vi "Bloco_escritaSuper.vi"(0 "reference":refnum<vi>, 1 "error in (no error)":errorcluster, 2 "Tag_para_PDF":string, 3 "Tipo de Dado":T6 items=["Engenharia", "Puro(mA)"], 4 "Abrir Editor Prioridade":bool, 7 "todos_os_dados_SAIDA":T1) -> (14 "reference out":refnum<vi>, 15 "error out":errorcluster)   [LabVIEW 2019]
uses:
  \\SERVERPC\Server/padrao_tipo_dado.ctl
  \\SERVERPC\Server/padrao_todos_os_dados_SAIDA.ctl
  \\SERVERPC\Server/padrao_UCM.004.EEL.0300_SAIDA.ctl
  \\SERVERPC\Server/padrao_UCM.004.EEL.0200_SAIDA.ctl
  \\SERVERPC\Server/padrao_INTERNO.ctl
  \\SERVERPC\Server/padrao_ADAM_SAIDA.ctl
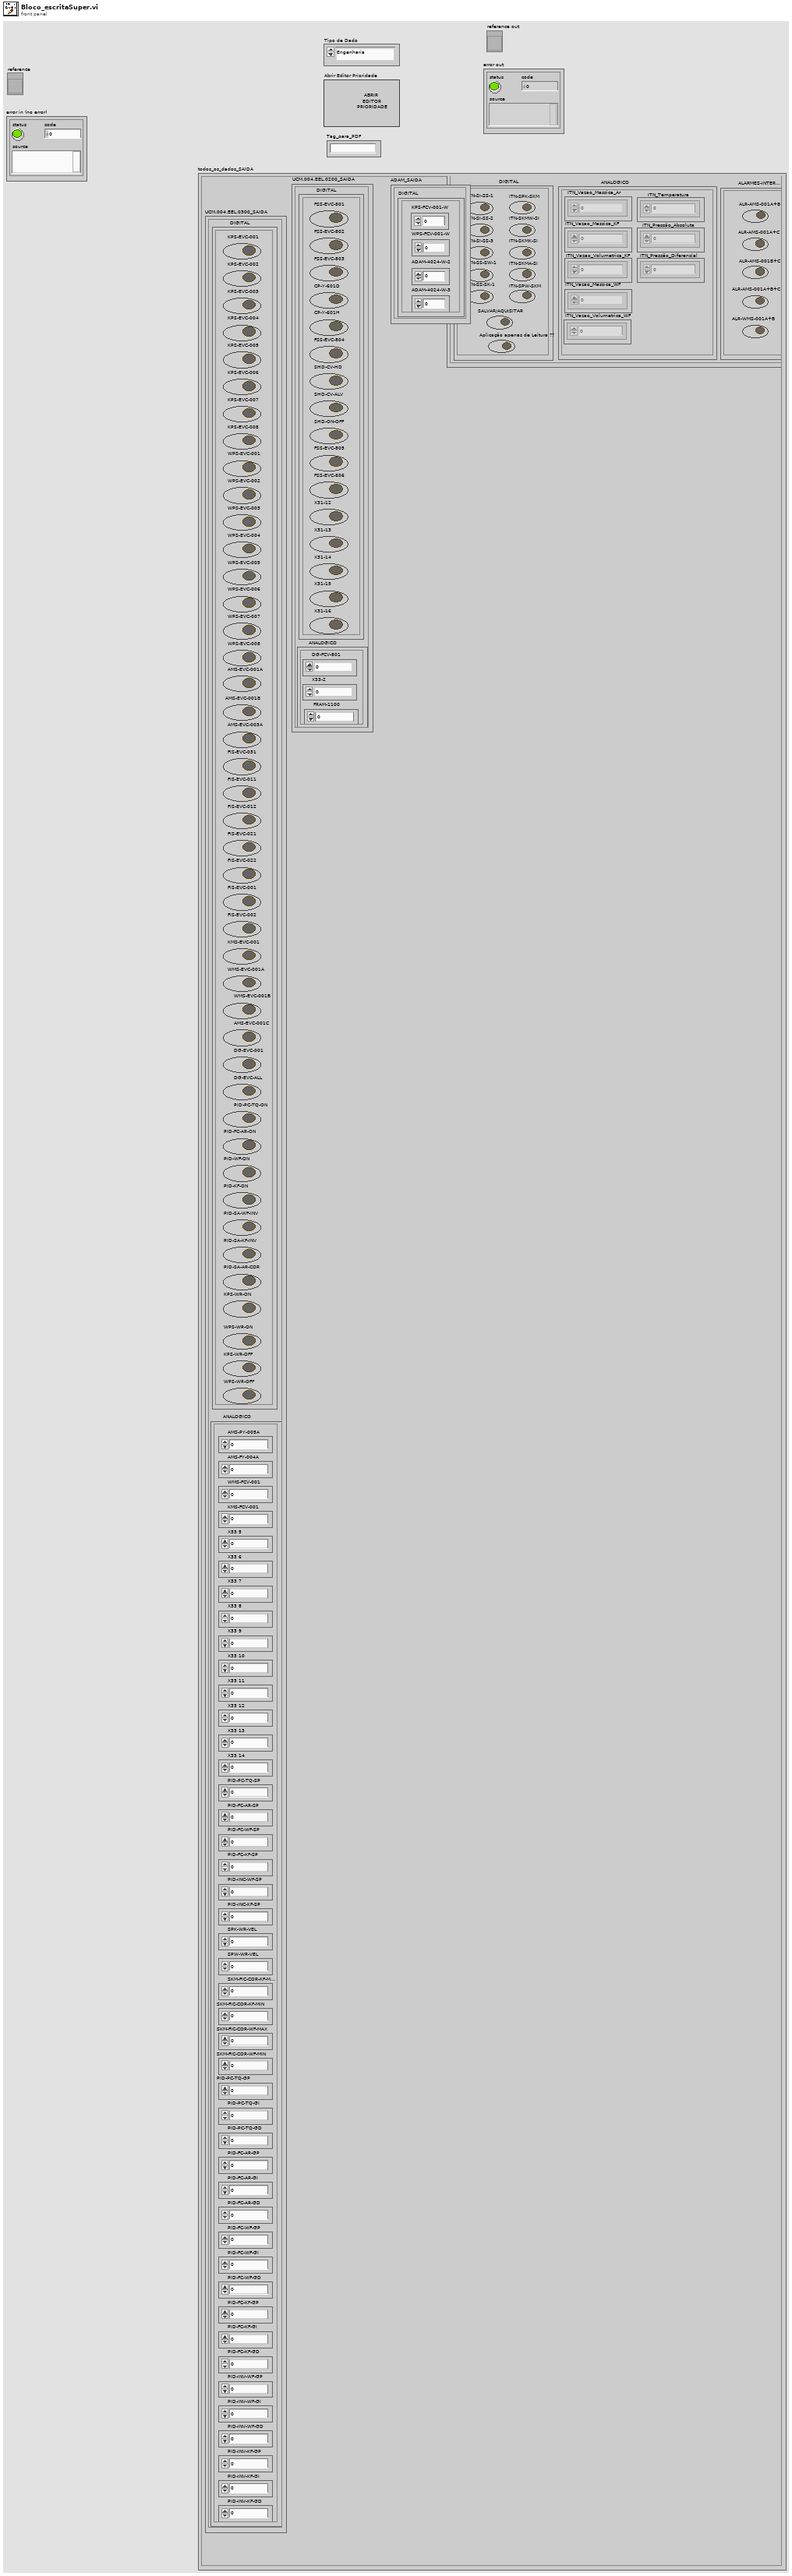
[diagram p1: front panel]
types:
  T1 = typedef "padrao_todos_os_dados_SAIDA.ctl" = cluster{"UCM.004.EEL.0300_SAIDA":T2, "UCM.004.EEL.0200_SAIDA":T3, "INTERNO":T4, "ADAM_SAIDA":T5}
  T2 = typedef "padrao_UCM.004.EEL.0300_SAIDA.ctl" = cluster{"DIGITAL":cluster{"KPS-EVC-001":bool, "KPS-EVC-002":bool, "KPS-EVC-003":bool, "KPS-EVC-004":bool, "KPS-EVC-005":bool, "KPS-EVC-006":bool, "KPS-EVC-007":bool, "KPS-EVC-008":bool, "WPS-EVC-001":bool, "WPS-EVC-002":bool, "WPS-EVC-003":bool, "WPS-EVC-004":bool, "WPS-EVC-005":bool, "WPS-EVC-006":bool, "WPS-EVC-007":bool, "WPS-EVC-008":bool, "AMS-EVC-001B":bool, "AMS-EVC-003A":bool, "FIS-EVC-031":bool, "FIS-EVC-011":bool, "FIS-EVC-012":bool, "FIS-EVC-021":bool, "FIS-EVC-022":bool, "FIS-EVC-001":bool, "FIS-EVC-002":bool, "KMS-EVC-001":bool, "WMS-EVC-001A":bool, "WMS-EVC-001B":bool, "AMS-EVC-001C":bool, "DG-EVC-001":bool, "DG-EVC-ALL":bool, "PID-PC-TQ-ON":bool, "PID-FC-AR-ON":bool, "PID-WF-ON":bool, "PID-KF-ON":bool, "PID-SA-WF-INV":bool, "PID-SA-KF-INV":bool, "PID-SA-AR-COR":bool, "KPS-WR-ON":bool, "WPS-WR-ON":bool, "KPS-WR-OFF":bool, "WPS-WR-OFF":bool, "AMS-EVC-001A":bool}, "ANALOGICO":cluster{"AMS-PY-005A":i16, "AMS-FY-004A":i16, "WMS-FCV-001":i16, "KMS-FCV-001":i16, "X33 5":i16, "X33 6":i16, "X33 7":i16, "X33 8":i16, "X33 9":i16, "X33 10":i16, "X33 11":i16, "X33 12":i16, "X33 13":i16, "X33 14":i16, "PID-PC-TQ-SP":i16, "PID-FC-AR-SP":i16, "PID-FC-WF-SP":i16, "PID-FC-KF-SP":i16, "PID-INC-WF-SP":i16, "PID-INC-KF-SP":i16, "SPK-WR-VEL":i32, "SPW-WR-VEL":i32, "SKM-FIC-COR-KF-MAX":dbl, "SKM-FIC-COR-KF-MIN":dbl, "SKM-FIC-COR-WF-MAX":dbl, "SKM-FIC-COR-WF-MIN":dbl, "PID-PC-TQ-GP":dbl, "PID-PC-TQ-GI":dbl, "PID-PC-TQ-GD":dbl, "PID-FC-AR-GP":dbl, "PID-FC-AR-GI":dbl, "PID-FC-AR-GD":dbl, "PID-FC-WF-GP":dbl, "PID-FC-WF-GI":dbl, "PID-FC-WF-GD":dbl, "PID-FC-KF-GP":dbl, "PID-FC-KF-GI":dbl, "PID-FC-KF-GD":dbl, "PID-INV-WF-GP":dbl, "PID-INV-WF-GI":dbl, "PID-INV-WF-GD":dbl, "PID-INV-KF-GP":dbl, "PID-INV-KF-GI":dbl, "PID-INV-KF-GD":dbl}}
  T3 = typedef "padrao_UCM.004.EEL.0200_SAIDA.ctl" = cluster{"DIGITAL":cluster{"FSS-EVC-801":bool, "FSS-EVC-802":bool, "FSS-EVC-803":bool, "CP-Y-601D":bool, "CP-Y-601H":bool, "FSS-EVC-804":bool, "SHD-CV-HD":bool, "SHD-CV-ALV":bool, "SHD-ON-OFF":bool, "FSS-EVC-805":bool, "FSS-EVC-806":bool, "X31-12":bool, "X31-13":bool, "X31-14":bool, "X31-15":bool, "X31-16":bool}, "ANALOGICO":cluster{"DG-FCV-801":i16, "X33-2":i16, "FRAM-1100":i16}}
  T4 = typedef "padrao_INTERNO.ctl" = cluster{"DIGITAL":cluster{"ITN-SI-SS-1":bool, "ITN-SI-SS-2":bool, "ITN-SI-SS-3":bool, "ITN-SS-SW-1":bool, "ITN-SS-SK-1":bool, "ITN-SPW-SKM":bool, "ITN-SKMW-SI":bool, "ITN-SKMK-SI":bool, "ITN-SKMA-SI":bool, "ITN-SPK-SKM":bool, "Aplicação apenas de Leitura ??":bool, "SALVAR/AQUISITAR":bool}, "ANALOGICO":cluster{"ITN_Vazao_Massica_Ar":dbl[], "ITN_Vazao_Volumetrica_WF":dbl[], "ITN_Vazao_Massica_KF":dbl[], "ITN_Vazao_Massica_WF":dbl[], "ITN_Vazao_Volumetrica_KF":dbl[], "ITN_Temperatura":dbl[], "ITN_Pressão_Absoluta":dbl[], "ITN_Pressão_Diferencial":dbl[]}, "ALARMES-INTERNOS":cluster{"ALR-AMS-001A+B":bool, "ALR-AMS-001A+C":bool, "ALR-AMS-001B+C":bool, "ALR-AMS-001A+B+C":bool, "ALR-WMS-001A+B":bool}}
  T5 = typedef "padrao_ADAM_SAIDA.ctl" = cluster{"DIGITAL":cluster{"KPS-FCV-001-W":dbl, "WPS-FCV-001-W":dbl, "ADAM-4024-W-2":dbl, "ADAM-4024-W-3":dbl}}
  T6 = typedef "padrao_tipo_dado.ctl" = u16
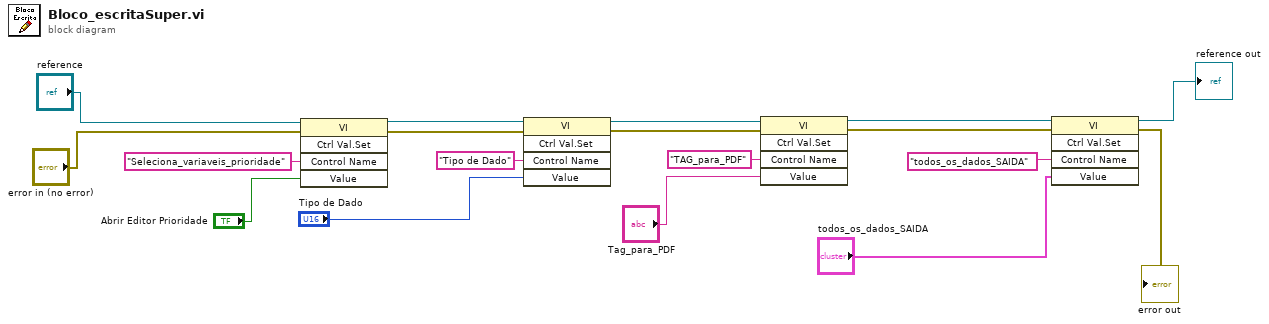
[diagram p0: block diagram]
diagram:
  n1 = invoke class="VI" method="Ctrl Val.Set"(reference="reference", error in="error in (no error)", "Control Name"="Seleciona_variaveis_prioridade", "Value"="Abrir Editor Prioridade") -> (reference out=w3:refnum<vi>, error out=w5:errorcluster)  [unwired: 1 in, 3 out]
  n2 = invoke class="VI" method="Ctrl Val.Set"(reference=w3, error in=w5, "Control Name"="Tipo de Dado", "Value"="Tipo de Dado") -> (reference out=w12:refnum<vi>, error out=w11:errorcluster)  [unwired: 1 in, 3 out]
  n3 = invoke class="VI" method="Ctrl Val.Set"(reference=w12, error in=w11, "Control Name"="TAG_para_PDF", "Value"="Tag_para_PDF") -> (reference out=w8:refnum<vi>, error out=w7:errorcluster)  [unwired: 1 in, 3 out]
  n4 = invoke class="VI" method="Ctrl Val.Set"(reference=w8, error in=w7, "Control Name"="todos_os_dados_SAIDA", "Value"="todos_os_dados_SAIDA") -> (reference out=→"reference out":refnum<vi>, error out=→"error out":errorcluster)  [unwired: 1 in, 3 out]
